vi "Dispersion measurements.vi"() -> ()   [LabVIEW 2015]
uses:
  <vilib>/express/express arith-compare/Formula/XNode/ExpressFormulaBlockNode.xnode
  <instrlib>/Rohde&Schwarz Vector Network Analyzer/Rohde&Schwarz Vector Network Analyzer.lvlib
panel:
  out "Run":i32
  in  "Minimum field (Oe)":dbl min=-1000.0 max=1000.0
  in  "Maximum field (Oe)":dbl=10.0 min=0.0 max=1000.0
  out "Amplifier LinMag gain":dbl
  in  "Power amplifier LinMag gain (if 0, it will be calculated)":dbl min=0.0 max=20.0
  in  "Stop frequency (Hz)":dbl=15000000000.0 min=0.0 max=20000000000.0
  in  "Start frequency (Hz)":dbl=100000.0 min=0.0 max=20000000000.0
  in  "1 Hz < IFBW < 1MHz (10 kHz default)":dbl=10000.0 min=1.0 max=10000000.0
  in  "-20 dB < Power < 20 dB (0 dB default)":dbl min=-20.0 max=20.0
  in  "Delay time along ther sample (ps)":dbl min=0.0 max=1000.0
  out "DMM reading":dbl=5.649249
  out "Current field point":i32=98
  in  "DMM's connection":refnum<visa-resource-name>="Multimeter"
  in  "Choose the folder where the field dependencies of S-parameters and Z will be saved":path=path "C:/Users/ZJUcomposite/Desktop/Tests/Stress-impedance measurements"
  in  "HMF's connection":refnum<visa-resource-name>="Generator"
  in  "VNA's connection":refnum<visa-resource-name>="ZNB-VNA"
  in  "Coil resistance > 0 (Ohm)":dbl=3.6 min=0.1 max=1000.0
  in  "Coil inductance > 0 (H)":dbl=0.0143 min=0.0 max=100.0
  in  "Number of field points":i32=20 min=2 max=1000 step=1
  in  "Volltage to field coefficient > 0 (Oe/V)":dbl=4.73 min=0.0 max=1000.0
  in  "Max input voltage for the amplifier (0<V<0.9)":dbl=0.5 min=0.0 max=10.0
  in  "Number of frequency points":i32=5000 min=3 max=20000
  in  "VNA's port(s) used for measurements":string(combo)="S21"
  # "The procedure measures the frequency dispersions of S-parameters and Z for the specified magnetic fields.\n\nVNA must be already calibrated before the measurements. The procedure will not change the calibration but you can   modify IFBW and power. The frequency measurement range must be within the calibration range. \n\nThe measured fields must be within the maximum (+/-) field range.\n\nThe voltage to field coefficient (Oe/V) must be found from the coil calibration.\n\nThe delay time along the sample must be found separately.\n\nThe coil resistance R and inductance L must be larger than zero. Measure them by a digital multimeter (DMM).\n\nPlease check the maximum input voltage max V allowed for your waveform amplifier. Also the ratio maxV / R must be below the current rate of your waveform amplifier.  \n\n******************************************\nDmitriy Makhnovskiy@Hangzhou December 2018\nSensing Materials Technology Ltd, UK\nE-mail: contact@sensmattech.co.uk"
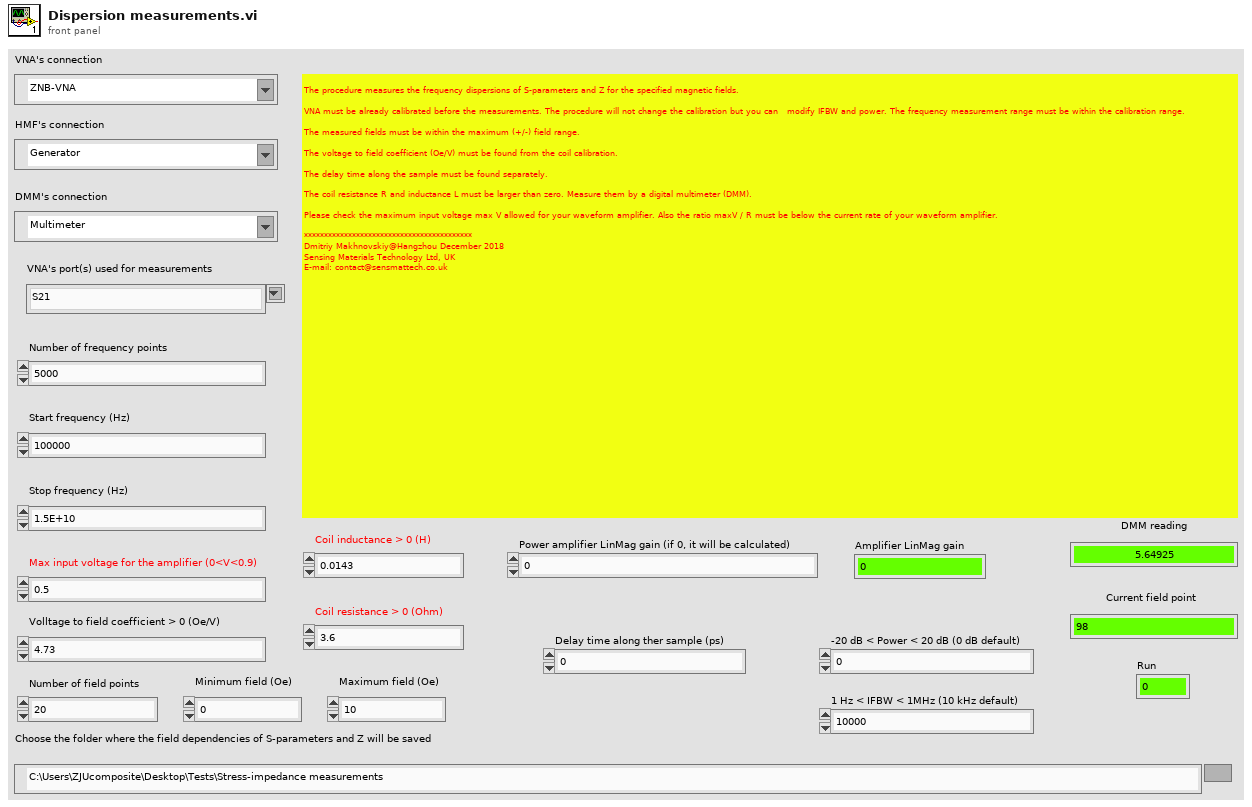
[diagram p1: front panel]
types:
  T1 = typedef "NI_Matrix.lvlib/RealMatrix.ctl" = dbl[][]
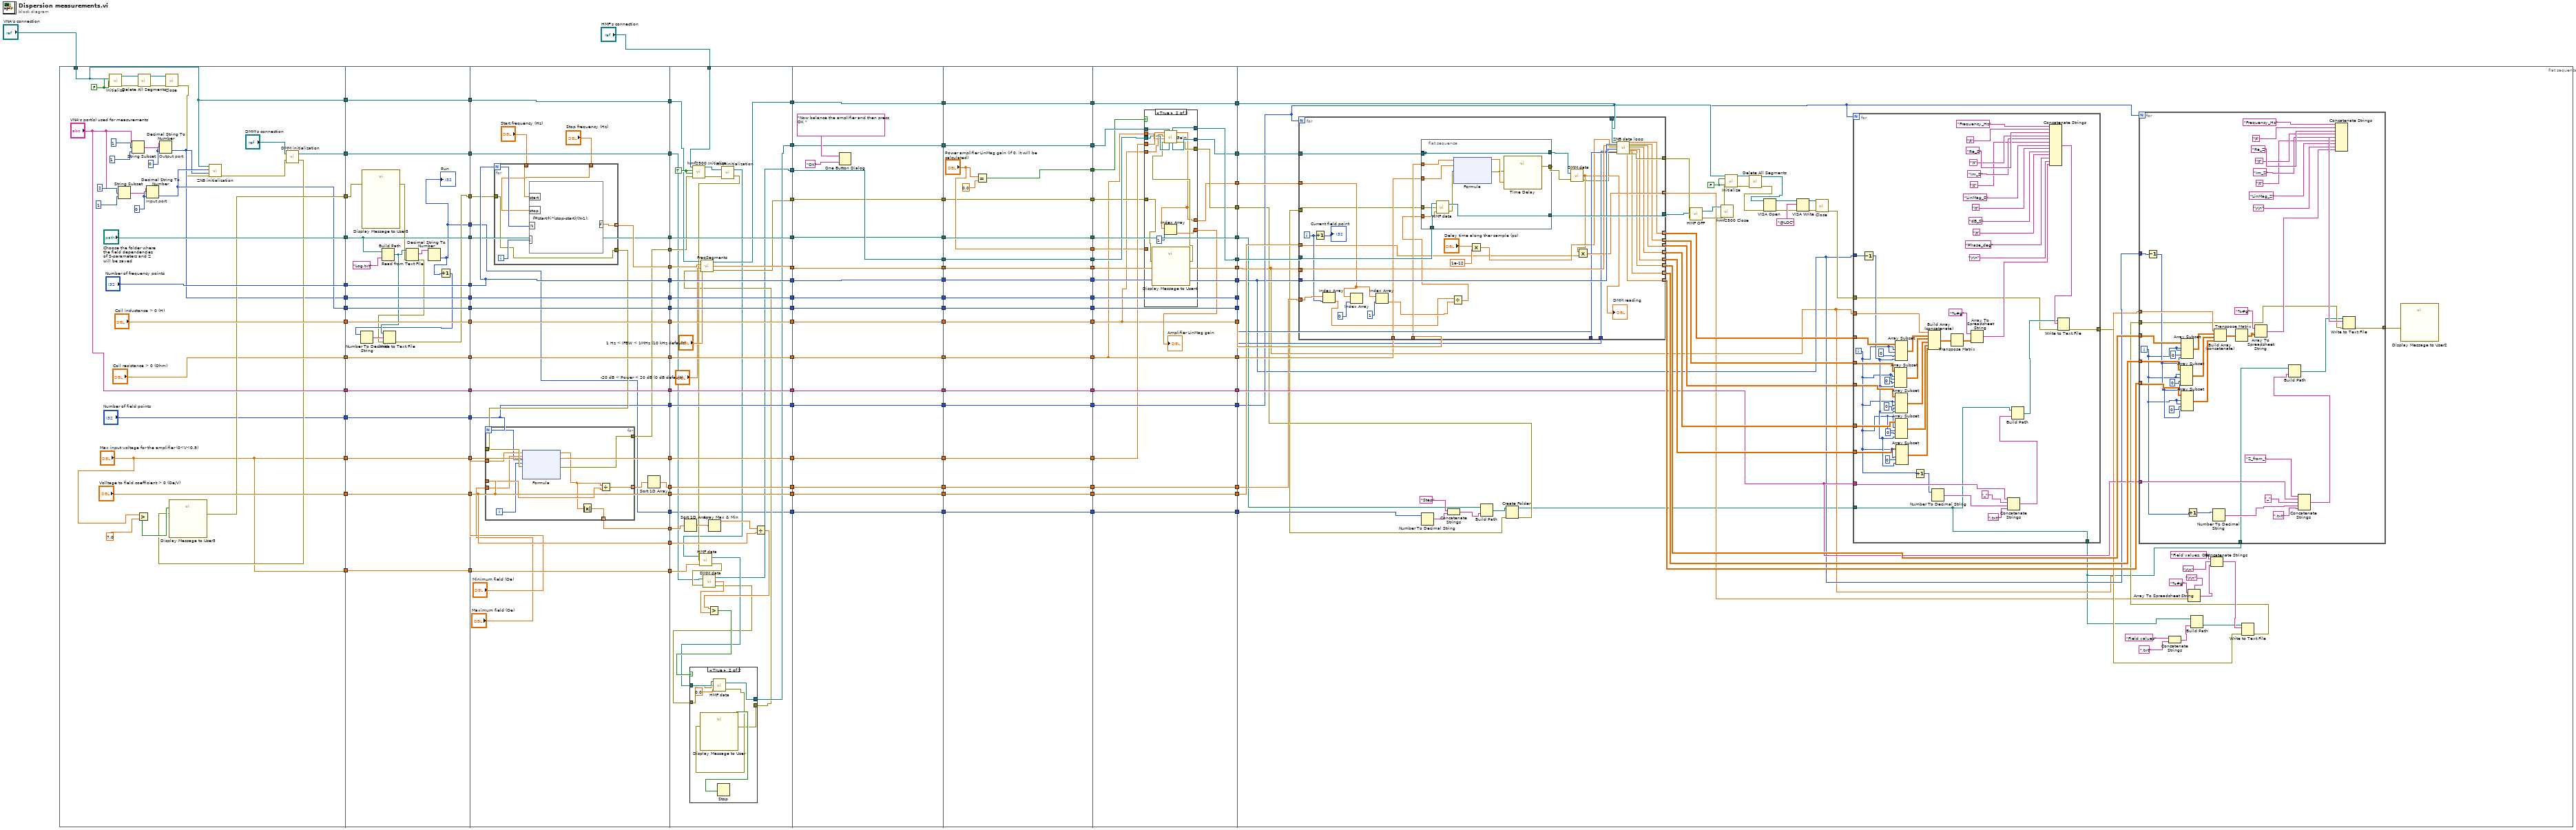
[diagram p0: block diagram]
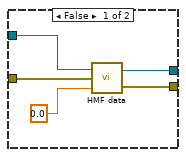
[diagram p2: hidden frame]
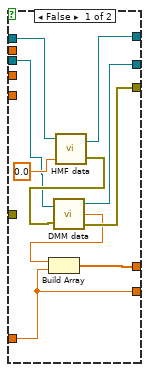
[diagram p3: hidden frame]
diagram:
  n1 = flat-sequence {
    tunnel: [w128] -> w34
    tunnel: ["VNA's port(s) used for measurements"] -> w32
    tunnel: "VNA's connection" -> [w128]
    tunnel: ["Number of frequency points"] -> w30
    tunnel: ["Coil inductance > 0 (H)"] -> w28
    tunnel: ["Coil resistance > 0 (Ohm)"] -> w26
    tunnel: ["Max input voltage for the amplifier (0<V<0.9)"] -> w24
    tunnel: ["Volltage to field coefficient > 0 (Oe/V)"] -> w22
    tunnel: ["Choose the folder where the field dependencies of S-parameters and Z will be saved"] -> w20
    tunnel: [w138] -> w18
    tunnel: [w133] -> w16
    tunnel: [w131] -> w14
    tunnel: [w130] -> w12
    tunnel: ["Number of field points"] -> w10
    tunnel: ["Max input voltage for the amplifier (0<V<0.9)"] -> w8
    tunnel: w34 -> [w175]
    tunnel: [w175] -> w33
    tunnel: w32 -> [w174]
    tunnel: [w174] -> w31
    tunnel: w30 -> [w173]
    tunnel: [w173] -> w29
    tunnel: w28 -> [w172]
    tunnel: [w172] -> w27
    tunnel: w26 -> [w171]
    tunnel: [w171] -> w25
    tunnel: w24 -> [w170]
    tunnel: [w170] -> w23
    tunnel: w22 -> [w169]
    tunnel: [w169] -> w21
    tunnel: w20 -> [w162]
    tunnel: [w162] -> w19
    tunnel: w18 -> [w154]
    tunnel: [w156] -> w17
    tunnel: w16 -> [w168]
    tunnel: [w168] -> w15
    tunnel: w14 -> [w167]
    tunnel: [w167] -> w13
    tunnel: w12 -> [w166]
    tunnel: [w166] -> w11
    tunnel: w10 -> [w165]
    tunnel: [w165] -> w9
    tunnel: w8 -> [w164]
    tunnel: [w164] -> w7
    tunnel: [w155] -> w1
    tunnel: [w200] -> w120
    tunnel: [w197] -> w118
    tunnel: [w179] -> w116
    tunnel: [w199] -> w113
    tunnel: w33 -> [w199]
    tunnel: [w198] -> w111
    tunnel: w31 -> [w198]
    tunnel: w29 -> [w197]
    tunnel: [w196] -> w108
    tunnel: w27 -> [w196]
    tunnel: [w195] -> w106
    tunnel: w25 -> [w195]
    tunnel: [w183] -> w104
    tunnel: w23 -> [w183]
    tunnel: [w181] -> w102
    tunnel: w21 -> [w181]
    tunnel: [w194] -> w100
    tunnel: w19 -> [w194]
    tunnel: w17 -> [w190]
    tunnel: [w193] -> w98
    tunnel: w15 -> [w193]
    tunnel: [w192] -> w96
    tunnel: w13 -> [w192]
    tunnel: [w191] -> w94
    tunnel: w11 -> [w191]
    tunnel: w9 -> [w186]
    tunnel: [w186] -> w92
    tunnel: [w184] -> w90
    tunnel: [w182] -> w89
    tunnel: [w181] -> w88
    tunnel: [w180] -> w87
    tunnel: w7 -> [w180]
    tunnel: [w176] -> w2
    tunnel: w1 -> [w176]
    tunnel: w120 -> [w259]
    tunnel: [w258] -> w119
    tunnel: w118 -> [w271]
    tunnel: [w271] -> w117
    tunnel: w116 -> [w239]
    tunnel: [w233] -> w115
    tunnel: [w257] -> w114
    tunnel: w113 -> [w241]
    tunnel: [w267] -> w112
    tunnel: w111 -> [w267]
    tunnel: "HMF's connection" -> [w240]
    tunnel: [w266] -> w109
    tunnel: w108 -> [w266]
    tunnel: [w265] -> w107
    tunnel: w106 -> [w265]
    tunnel: [w264] -> w105
    tunnel: w104 -> [w264]
    tunnel: [w263] -> w103
    tunnel: w102 -> [w263]
    tunnel: [w262] -> w101
    tunnel: w100 -> [w262]
    tunnel: [w243] -> w99
    tunnel: w98 -> [w235]
    tunnel: [w261] -> w97
    tunnel: w96 -> [w261]
    tunnel: [w260] -> w95
    tunnel: w94 -> [w260]
    tunnel: [w254] -> w93
    tunnel: w92 -> [w254]
    tunnel: [w253] -> w91
    tunnel: w90 -> [w253]
    tunnel: w89 -> [w250]
    tunnel: w88 -> [w249]
    tunnel: w87 -> [w247]
    tunnel: [w237] -> w37
    tunnel: [w231] -> w3
    tunnel: w2 -> [w231]
    tunnel: w119 -> [w300]
    tunnel: [w300] -> w70
    tunnel: w117 -> [w299]
    tunnel: [w299] -> w68
    tunnel: w115 -> [w298]
    tunnel: [w298] -> w66
    tunnel: [w297] -> w64
    tunnel: w114 -> [w297]
    tunnel: [w296] -> w62
    tunnel: w112 -> [w296]
    tunnel: [w295] -> w60
    tunnel: w109 -> [w295]
    tunnel: [w294] -> w58
    tunnel: w107 -> [w294]
    tunnel: [w293] -> w56
    tunnel: w105 -> [w293]
    tunnel: [w292] -> w54
    tunnel: w103 -> [w292]
    tunnel: [w291] -> w52
    tunnel: w101 -> [w291]
    tunnel: [w290] -> w50
    tunnel: w99 -> [w290]
    tunnel: [w289] -> w48
    tunnel: w97 -> [w289]
    tunnel: [w288] -> w46
    tunnel: w95 -> [w288]
    tunnel: [w287] -> w44
    tunnel: w93 -> [w287]
    tunnel: [w286] -> w42
    tunnel: w91 -> [w286]
    tunnel: w37 -> [w285]
    tunnel: [w285] -> w36
    tunnel: [w284] -> w4
    tunnel: w3 -> [w284]
    tunnel: w70 -> [w322]
    tunnel: [w322] -> w69
    tunnel: w68 -> [w321]
    tunnel: [w321] -> w67
    tunnel: w66 -> [w320]
    tunnel: [w320] -> w65
    tunnel: w64 -> [w319]
    tunnel: [w319] -> w63
    tunnel: w62 -> [w318]
    tunnel: [w318] -> w61
    tunnel: w60 -> [w317]
    tunnel: [w317] -> w59
    tunnel: w58 -> [w316]
    tunnel: [w316] -> w57
    tunnel: w56 -> [w315]
    tunnel: [w315] -> w55
    tunnel: w54 -> [w314]
    tunnel: [w314] -> w53
    tunnel: w52 -> [w313]
    tunnel: [w313] -> w51
    tunnel: w50 -> [w312]
    tunnel: [w312] -> w49
    tunnel: w48 -> [w311]
    tunnel: [w311] -> w47
    tunnel: w46 -> [w310]
    tunnel: [w310] -> w45
    tunnel: w44 -> [w309]
    tunnel: [w309] -> w43
    tunnel: w42 -> [w308]
    tunnel: [w308] -> w41
    tunnel: [w306] -> w40
    tunnel: ["Power amplifier LinMag gain (if 0, it will be calculated)"] -> w39
    tunnel: w36 -> [w304]
    tunnel: [w304] -> w35
    tunnel: [w303] -> w5
    tunnel: w4 -> [w303]
    tunnel: w69 -> [w346]
    tunnel: [w346] -> w86
    tunnel: w67 -> [w345]
    tunnel: [w345] -> w85
    tunnel: w65 -> [w335]
    tunnel: [w333] -> w84
    tunnel: w63 -> [w344]
    tunnel: [w344] -> w83
    tunnel: w61 -> [w343]
    tunnel: [w343] -> w82
    tunnel: w59 -> [w325]
    tunnel: [w325] -> w81
    tunnel: w57 -> [w324]
    tunnel: [w324] -> w80
    tunnel: w55 -> [w334]
    tunnel: w53 -> [w342]
    tunnel: [w342] -> w79
    tunnel: w51 -> [w341]
    tunnel: [w341] -> w78
    tunnel: w49 -> [w336]
    tunnel: [w328] -> w77
    tunnel: w47 -> [w340]
    tunnel: [w340] -> w76
    tunnel: w45 -> [w339]
    tunnel: [w339] -> w75
    tunnel: w43 -> [w338]
    tunnel: [w338] -> w74
    tunnel: w41 -> [w337]
    tunnel: [w337] -> w73
    tunnel: [w332] -> w72
    tunnel: [w331] -> w71
    tunnel: w40 -> [w329]
    tunnel: w39 -> [w327]
    tunnel: w35 -> [w326]
    tunnel: [w323] -> w6
    tunnel: w5 -> [w323]
    tunnel: w86 -> [w393]
    tunnel: w85 -> [w394]
    tunnel: w84 -> [w431]
    tunnel: w83 -> [w422]
    tunnel: w82 -> [w410]
    tunnel: w81 -> [w408]
    tunnel: w80 -> [w407]
    tunnel: w79 -> [w406]
    tunnel: w78 -> [w374]
    tunnel: w77 -> [w405]
    tunnel: w76 -> [w403]
    tunnel: w75 -> [w402]
    tunnel: w74 -> [w395]
    tunnel: w73 -> [w397]
    tunnel: w72 -> [w373]
    tunnel: w71 -> [w396]
    tunnel: w6 -> [w377]
    frame #0 {
      w144 = FALSE
      w152 = 0
      w148 = 0
      n2 = call <instrlib>:"Initialize.vi"("VISA resource name"=w128, "ID Query (T: Check)"=w144, "Reset (T: Reset)"=w144) -> ("VISA resource name out"=w124:refnum<visa-resource-name>, "error out"=w126:errorcluster)  [unwired: 11 in]
      n3 = String Subset(string="VNA's port(s) used for measurements", offset (0)=2, length (rest)=1) -> (substring=w151:string)
      n4 = String Subset(string="VNA's port(s) used for measurements", offset (0)=1, length (rest)=1) -> (substring=w147:string)
      n5 = Greater?(x="Max input voltage for the amplifier (0<V<0.9)", y=7.0) -> (0:w136:bool)
      n6 = call <instrlib>:"Delete All Segments.vi"("error in (no error)"=w126, "VISA resource name"=w124) -> ("error out"=w125:errorcluster, "VISA resource name out"=w123:refnum<visa-resource-name>)  [unwired: 8 in]
      n7 = Decimal String To Number "Input port"(string=w151, offset=w152, default (0L)=w152) -> (number=w131:i32)  [unwired: 1 out]
      n8 = Decimal String To Number "Output port"(string=w147, offset=w148, default (0L)=w148) -> (number=w130:i32)  [unwired: 1 out]
      n9 = call <instrlib>:"Close.vi"("error in (no error)"=w125, "VISA resource name"=w123) -> ("error out"=w127:errorcluster)  [unwired: 9 in]
      n10 = call "ZNB initialization.vi"("error in (no error)"=w127, "Output port"=w130, "Input port"=w131, "VISA resource name"=w128) -> ("error out"=w129:errorcluster)  [unwired: 7 in]
      n11 = call "DMM initialization.vi"("error in (no error)"=w129, "VISA resource name"="DMM's connection") -> ("error out"=w132:errorcluster, "VISA resource name out"=w133:refnum<visa-resource-name>)
      n12 = call "Display Message to User3"("error in (no error)"=w132, "Enable"=w136) -> ("error out"=w138:errorcluster)  [unwired: 8 in, 1 out]
    }
    frame #1 {
      n13 = call "Display Message to User5"("error in (no error)"=w154) -> ("error out"=w153:errorcluster)  [unwired: 9 in, 1 out]
      n14 = Build Path(base path=w162, name or relative path="Log.txt") -> (appended path=w159:path)
      n15 = Read from Text File(file (use dialog)=w159, error in=w153) -> (text=w161:string, error out=w157:errorcluster)  [unwired: 2 in, 2 out]
      n16 = Decimal String To Number(string=w161) -> (number=w155:i32)  [unwired: 2 in, 1 out]
      "Run" <- w155
      n17 = Increment(x=w155) -> (x+1=w158:i32)
      n18 = Number To Decimal String(number=w158) -> (decimal integer string=w160:string)  [unwired: 1 in]
      n19 = Write to Text File(file (use dialog)=w159, text=w160, error in=w157) -> (error out=w156:errorcluster)  [unwired: 1 in, 2 out]
    }
    frame #2 {
      n20 = for {
        N: w197 -> [w229]
        tunnel: [w228] -> w200 mode=indexing
        tunnel: w190 -> [w225]
        tunnel: "Start frequency (Hz)" -> [w227]
        tunnel: "Stop frequency (Hz)" -> [w226]
        tunnel: [w225] -> w187
        i -> [w230]
        n21 = formula code="f=start+i*(stop-start)/(N-1);"("start"=w227, "stop"=w226, "N"=w229, "i"=w230) -> ("f"=w228:dbl)
      }
      n22 = for {
        N: w186 -> [w202]
        tunnel: w187 -> [w207]
        tunnel: w181 -> [w210]
        tunnel: [w209] -> w185 mode=indexing
        tunnel: [w208] -> w182 mode=indexing
        tunnel: [w206] -> w179
        tunnel: "Minimum field (Oe)" -> [w204]
        tunnel: "Maximum field (Oe)" -> [w203]
        i -> [w201]
        n23 = xnode "Formula"("Min"=w204, "Max"=w203, "N"=w202, "i"=w201, "error in (no error)"=w207) -> ("Result"=w205:dbl, "error out"=w206:errorcluster)
        n24 = Absolute Value(x=w205) -> (abs(x)=w208:dbl)
        n25 = Divide(x=w205, y=w210) -> (x/y=w209:ext)
      }
      n26 = Sort 1D Array(array=w185) -> (sorted array=w184:ext[])
    }
    frame #3 {
      w270 = TRUE
      n27 = Sort 1D Array(array=w250) -> (sorted array=w251:dbl[])
      n28 = call <instrlib>:"hmf2500 Initialize.vi"("error in (no error)"=w239, "Reset (Reset)"=w270, "ID Query (Check)"=w270, "VISA resource name"=w240) -> ("error out"=w268:errorcluster, "VISA resource name out"=w269:refnum<visa-resource-name>)  [unwired: 6 in]
      n29 = Array Max & Min(array=w251) -> (max value=w252:dbl)  [unwired: 3 out]
      n30 = call "HMF initialization.vi"("error in (no error)"=w268, "VISA resource name"=w269) -> ("error out"=w248:errorcluster, "VISA resource name out"=w242:refnum<visa-resource-name>)
      n31 = call "HMF data.vi"("DC offset"=w247, "error in (no error)"=w248, "VISA resource name"=w242) -> ("error out"=w236:errorcluster, "VISA resource name out"=w244:refnum<visa-resource-name>)
      n32 = call "DMM data.vi"("VISA resource name"=w235, "error in (no error)"=w236) -> ("VISA resource name out"=w233:refnum<visa-resource-name>, "Voltage"=w234:dbl, "error out"=w232:errorcluster)
      n33 = Divide(x=w252, y=w249) -> (x/y=w246:dbl)
      n34 = Greater?(x=w246, y=w234) -> (0:w245:bool)
      n35 = case shown="True" w245 {
        tunnel: w244 -> [w275 w283]
        tunnel: w232 -> [w272 w280]
        tunnel: [w274 w277] -> w243
        tunnel: [w273 w278] -> w238
        frame False {
          n36 = call "HMF data.vi"("DC offset"=0.0, "error in (no error)"=w272, "VISA resource name"=w275) -> ("error out"=w273:errorcluster, "VISA resource name out"=w274:refnum<visa-resource-name>)
        }
        frame True {
          n37 = call "HMF data.vi"("DC offset"=0.0, "error in (no error)"=w280, "VISA resource name"=w283) -> ("error out"=w279:errorcluster, "VISA resource name out"=w277:refnum<visa-resource-name>)
          n38 = call "Display Message to User"("error in (no error)"=w279) -> ("error out"=w278:errorcluster, "OK"=w281:bool)  [unwired: 9 in]
          n39 = Stop(stop? (T)=w281) -> ()
        }
      }
      n40 = call "FreqSegments.vi"("VISA resource name"=w241, "FrequenciesIn"=w259, "Power"="-20 dB < Power < 20 dB (0 dB default)", "error in (no error)"=w238, "IFBW"="1 Hz < IFBW < 1MHz (10 kHz default)") -> ("VISA resource name out"=w257:refnum<visa-resource-name>, "FrequenciesOut"=w258:dbl[], "error out"=w237:errorcluster)
    }
    frame #4 {
      n41 = One Button Dialog(message="Now balance the amplifier and then press OK ", button name ("OK")="OK") -> ()  [unwired: 1 out]
    }
    frame #5 {
      n42 = Equal?(x="Power amplifier LinMag gain (if 0, it will be calculated)", y=0.0) -> (x = y?=w306:bool)
    }
    frame #6 {
      n43 = case shown="True" w329 {
        tunnel: w336 -> [w355 w366]
        tunnel: w335 -> [w352 w364]
        tunnel: w334 -> [_ w367]
        tunnel: [w354 w365] -> w333
        tunnel: [w351 w363] -> w328
        tunnel: [w350 w362] -> w332
        tunnel: [w347 w360] -> w331
        tunnel: [w348 w359] -> w330
        tunnel: w327 -> [w348 _]
        tunnel: w326 -> [_ w368]
        tunnel: w325 -> [_ w358]
        tunnel: w324 -> [_ w357]
        frame False {
          n44 = call "HMF data.vi"("DC offset"=0.0, "VISA resource name"=w355) -> ("error out"=w353:errorcluster, "VISA resource name out"=w354:refnum<visa-resource-name>)  [unwired: 1 in]
          n45 = call "DMM data.vi"("VISA resource name"=w352, "error in (no error)"=w353) -> ("VISA resource name out"=w351:refnum<visa-resource-name>, "Voltage"=w349:dbl, "error out"=w350:errorcluster)
          n46 = Build Array(w349, w348) -> (w347:dbl[])
        }
        frame True {
          n47 = call "Display Message to User4"("error in (no error)"=w368) -> ("error out"=w361:errorcluster)  [unwired: 9 in, 1 out]
          n48 = call "Gain.vi"("DMM VISA in"=w364, "HMF VISA in"=w366, "error in (no error)"=w361, "R"=w357, "L"=w358, "Max v input"=w367) -> ("error out"=w362:errorcluster, "Polynomial coeff"=w360:dbl[], "DMM VISA out"=w363:refnum<visa-resource-name>, "HMF VISA out"=w365:refnum<visa-resource-name>)  [unwired: 2 in]
          n49 = Index Array(array=w360, index=1) -> (element=w359:dbl)
        }
      }
      "Amplifier LinMag gain" <- w330
    }
    frame #7 {
      w420 = FALSE
      n50 = Number To Decimal String(number=w377) -> (decimal integer string=w379:string)  [unwired: 1 in]
      n51 = Concatenate Strings("Step", w379) -> (w375:string)
      n52 = Build Path(base path=w374, name or relative path=w375) -> (appended path=w376:path)
      n53 = Create Folder(path (use dialog)=w376, error in=w373) -> (created path=w371:path, error out=w372:errorcluster)  [unwired: 1 in, 1 out]
      n54 = for {
        N: w395 -> [_]
        tunnel: w406 -> [w524]
        tunnel: w394 -> [w549]
        tunnel: [w545] -> w380 mode=indexing
        tunnel: w431 -> [w552]
        tunnel: [w551] -> w430
        tunnel: w422 -> [w550]
        tunnel: w393 -> [w548]
        tunnel: [w546] -> w411 mode=indexing
        tunnel: [w547] -> w404
        tunnel: [w544] -> w412 mode=indexing
        tunnel: [w543] -> w413 mode=indexing
        tunnel: [w542] -> w414 mode=indexing
        tunnel: [w541] -> w415 mode=indexing
        tunnel: [w540] -> w416 mode=indexing
        tunnel: [w539] -> w417 mode=indexing
        tunnel: [w538] -> w418 mode=indexing
        tunnel: w408 -> [w537]
        tunnel: w407 -> [w536]
        tunnel: w405 -> [w518]
        tunnel: w403 -> [w535]
        tunnel: w402 -> [w534]
        tunnel: w397 -> [w529]
        tunnel: w396 -> [w526]
        tunnel: w372 -> [w515]
        i -> [w528]
        n55 = Increment(x=w528) -> (x+1=→"Current field point":i32)
        n56 = Index Array(array=w529, index=w528) -> (element=w516:ext)
        n57 = Index Array(array=w526, index=0) -> ()  [unwired: 1 out]
        n58 = Index Array(array=w526, index=1) -> (element=w519:dbl)
        n59 = flat-sequence {
          tunnel: [w563] -> w551
          tunnel: w552 -> [w560]
          tunnel: [w559] -> w522
          tunnel: w537 -> [w558]
          tunnel: w536 -> [w557]
          tunnel: w515 -> [w555]
          tunnel: w523 -> [w554]
          tunnel: [w553] -> _
          tunnel: w518 -> [w553]
          tunnel: [w553] -> w517
          frame #0 {
            n60 = call "HMF data.vi"("DC offset"=w554, "error in (no error)"=w555, "VISA resource name"=w560) -> ("error out"=w556:errorcluster, "VISA resource name out"=w563:refnum<visa-resource-name>)
            n61 = xnode "Formula"("X1"=w558, "X2"=w557, "error in (no error)"=w556) -> ("Result"=w562:dbl, "error out"=w561:errorcluster)
            n62 = call "Time Delay"("error in (no error)"=w561, "Delay Time (s)"=w562) -> ("error out"=w559:errorcluster)  [unwired: 9 in]
          }
        }
        n63 = Divide(x=w516, y=w519) -> (x/y=w523:ext)
        n64 = Multiply(x="Delay time along ther sample (ps)", y=1e-12) -> (x*y=w531:dbl)
        n65 = call "DMM data.vi"("VISA resource name"=w517, "error in (no error)"=w522) -> ("Voltage"=w521:dbl, "error out"=w520:errorcluster)  [unwired: 1 out]
        "DMM reading" <- w521
        n66 = Multiply(x=w521, y=w524) -> (x*y=w545:ext)
        n67 = call "ZNB data loop.vi"("VISA resource name"=w550, "Number of frequency points"=w549, "Frequencies"=w548, "Delay Time"=w531, "Output Port"=w534, "Input Port"=w535, "error in (no error)"=w520) -> ("error out"=w547:errorcluster, "ReS"=w538:dbl[], "ImS"=w539:dbl[], "LinMagS"=w540:dbl[], "dBS"=w541:dbl[], "Phase"=w542:dbl[], "ReZ"=w543:dbl[], "ImZ"=w544:dbl[], "LinMagZ"=w546:dbl[])  [unwired: 12 in]
      }
      n68 = call "HMF OFF.vi"("error in (no error)"=w404, "VISA resource name"=w430) -> ("error out"=w428:errorcluster, "VISA resource name out"=w429:refnum<visa-resource-name>)
      n69 = call <instrlib>:"hmf2500 Close.vi"("error in (no error)"=w428, "VISA resource name"=w429) -> ("error out"=w421:errorcluster)  [unwired: 9 in]
      n70 = call <instrlib>:"Initialize.vi"("VISA resource name"=w422, "ID Query (T: Check)"=w420, "Reset (T: Reset)"=w420, "error in (no error)"=w421) -> ("VISA resource name out"=w400:refnum<visa-resource-name>, "error out"=w401:errorcluster)  [unwired: 10 in]
      n71 = call <instrlib>:"Delete All Segments.vi"("error in (no error)"=w401, "VISA resource name"=w400) -> ("error out"=w399:errorcluster, "VISA resource name out"=w398:refnum<visa-resource-name>)  [unwired: 8 in]
      n72 = VISA Open(error in (no error)=w399, VISA resource name=w398) -> (VISA resource name=w424:refnum<visa-resource-name>, error out=w423:errorcluster)  [unwired: 3 in]
      n73 = VISA Write(VISA resource name=w424, write buffer="@LOC", error in (no error)=w423) -> (VISA resource name out=w426:refnum<visa-resource-name>, error out=w425:errorcluster)  [unwired: 1 out]
      n74 = call <instrlib>:"Close.vi"("error in (no error)"=w425, "VISA resource name"=w426) -> ("error out"=w419:errorcluster)  [unwired: 9 in]
      n75 = for {
        N: w395 -> [_]
        tunnel: w419 -> [w470]
        tunnel: w418 -> [w514]
        tunnel: w393 -> [w513]
        tunnel: w394 -> [w511]
        tunnel: w410 -> [w487]
        tunnel: w417 -> [w504]
        tunnel: w416 -> [w502]
        tunnel: w415 -> [w500]
        tunnel: w414 -> [w498]
        tunnel: [w473] -> w382
        tunnel: [w469] -> w370
        tunnel: w371 -> [w469]
        i -> [w477]
        n76 = Decrement(x=w511) -> (x-1=w481:i32)
        n77 = Array Subset(array=w504, index (row)=w477, length (row)=w477, index (col)=0, length (col)=w481) -> (w505:dbl[][])
        n78 = Array Subset(array=w514, index (row)=w477, length (row)=w477, index (col)=0, length (col)=w481) -> (w479:dbl[][])
        n79 = Array Subset(array=w502, index (row)=w477, length (row)=w477, index (col)=0, length (col)=w481) -> (w503:dbl[][])
        n80 = Array Subset(array=w500, index (row)=w477, length (row)=w477, index (col)=0, length (col)=w481) -> (w501:dbl[][])
        n81 = Array Subset(array=w498, index (row)=w477, length (row)=w477, index (col)=0, length (col)=w481) -> (w499:dbl[][])
        n82 = Increment(x=w477) -> (x+1=w476:i32)
        n83 = Build Array (concatenate)(w513, w479, w505, w503, w501, w499) -> (w480:T1)
        n84 = Number To Decimal String(number=w476) -> (decimal integer string=w474:string)  [unwired: 1 in]
        n85 = Transpose Matrix(1:w480) -> (0:w478:T1)
        n86 = Array To Spreadsheet String(array=w478, 3:"%#g") -> (spreadsheet string=w488:string)  [unwired: 1 in]
        n87 = Concatenate Strings(w487, "_", w474, ".txt") -> (w472:string)
        n88 = Build Path(base path=w469, name or relative path=w472) -> (appended path=w471:path)
        n89 = Concatenate Strings("Frequency_Hz", "\t", "Re_S", "\t", "Im_S", "\t", "LinMag_S", "\t", "dB_S", "\t", "Phase_deg", "\r\n", w488) -> (w509:string)
        n90 = Write to Text File(file (use dialog)=w471, text=w509, error in=w470) -> (error out=w473:errorcluster)  [unwired: 1 in, 2 out]
      }
      n91 = Concatenate Strings("Field values", ".txt") -> (w392:string)
      n92 = Array To Spreadsheet String(delimiter (Tab)="\r\n", array=w380, 3:"%#g") -> (spreadsheet string=w384:string)
      n93 = Build Path(base path=w370, name or relative path=w392) -> (appended path=w387:path)
      n94 = Concatenate Strings("Field values, Oe", "\r\n", w384) -> (w389:string)
      n95 = Write to Text File(file (use dialog)=w387, text=w389, error in=w382) -> (error out=w381:errorcluster)  [unwired: 1 in, 2 out]
      n96 = for {
        N: w395 -> [_]
        tunnel: w413 -> [w468]
        tunnel: w393 -> [w467]
        tunnel: w394 -> [w465]
        tunnel: w410 -> [w449]
        tunnel: [w459] -> w409
        tunnel: w412 -> [w457]
        tunnel: w411 -> [w455]
        tunnel: w381 -> [w441]
        tunnel: w370 -> [w432]
        i -> [w438]
        n97 = Decrement(x=w465) -> (x-1=w442:i32)
        n98 = Array Subset(array=w457, index (row)=w438, length (row)=w438, index (col)=0, length (col)=w442) -> (w458:dbl[][])
        n99 = Array Subset(array=w468, index (row)=w438, length (row)=w438, index (col)=0, length (col)=w442) -> (w466:dbl[][])
        n100 = Array Subset(array=w455, index (row)=w438, length (row)=w438, index (col)=0, length (col)=w442) -> (w456:dbl[][])
        n101 = Increment(x=w438) -> (x+1=w437:i32)
        n102 = Number To Decimal String(number=w437) -> (decimal integer string=w436:string)  [unwired: 1 in]
        n103 = Build Array (concatenate)(w467, w466, w458, w456) -> (w440:T1)
        n104 = Transpose Matrix(1:w440) -> (0:w439:T1)
        n105 = Array To Spreadsheet String(array=w439, 3:"%#g") -> (spreadsheet string=w446:string)  [unwired: 1 in]
        n106 = Concatenate Strings("Z_from_", w449, "_", w436, ".txt") -> (w434:string)
        n107 = Build Path(base path=w432, name or relative path=w434) -> (appended path=w433:path)
        n108 = Concatenate Strings("Frequency_Hz", "\t", "Re_Z", "\t", "Im_Z", "\t", "LinMag_Z", "\r\n", w446) -> (w463:string)
        n109 = Write to Text File(file (use dialog)=w433, text=w463, error in=w441) -> (error out=w459:errorcluster)  [unwired: 1 in, 2 out]
      }
      n110 = call "Display Message to User2"("error in (no error)"=w409) -> ()  [unwired: 9 in, 2 out]
    }
  }
